vi "Requests.vi"(8 "error in (no error)":errorcluster, 9 "write enable":bool=TRUE, 10 "msg":refnum<queue>, 11 "SP in":refnum<class "Save messages PGserver.lvclass">) -> (0 "error out":errorcluster, 1 "queue deleted":bool, 3 "SP out":refnum<class "Save messages PGserver.lvclass">)   [LabVIEW 2019, in "Save messages PGserver.lvclass"]
uses:
  Save messages PGserver.lvclass
  Save messages PGserver.lvclass/Save messages PGserver.ctl
  PostgreSQL2LabVIEW/libpqlv/src/PQresultErrorMessage.vi
  PostgreSQL2LabVIEW/libpqUtility/src/PQclear.vi
  PostgreSQL2LabVIEW/libpqlv/src/PQsendQuery.vi
  PostgreSQL2LabVIEW/libpqlv/src/PQgetResult.vi
  PostgreSQL2LabVIEW/libpqlv/src/PQresultStatus.vi
  PostgreSQL2LabVIEW/libpqlv/src/PQclear.vi
  PostgreSQL2LabVIEW/libpqUtility/libpqutility.lvlib
  PostgreSQL2LabVIEW/libpqUtility64/libpqutility64.lvlib
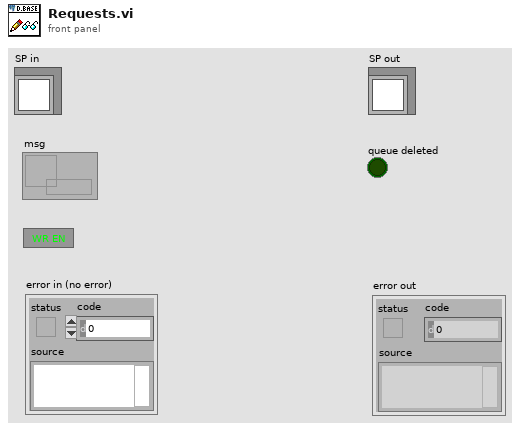
[diagram p1: front panel]
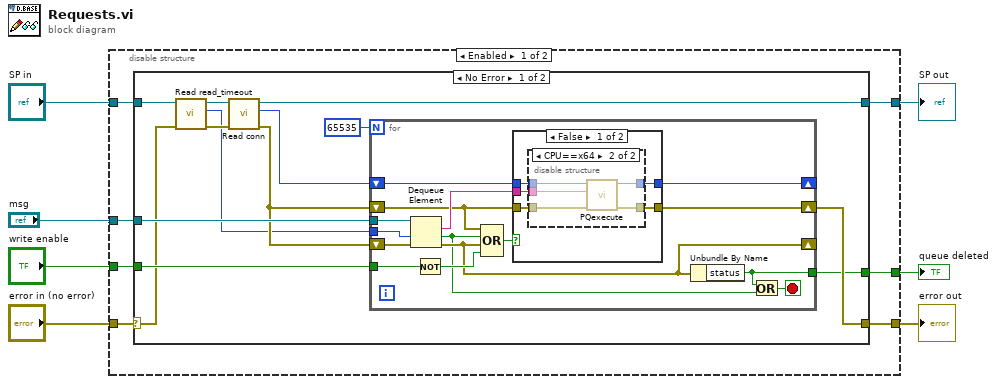
[diagram p0: block diagram]
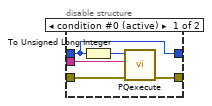
[diagram p2: hidden frame]
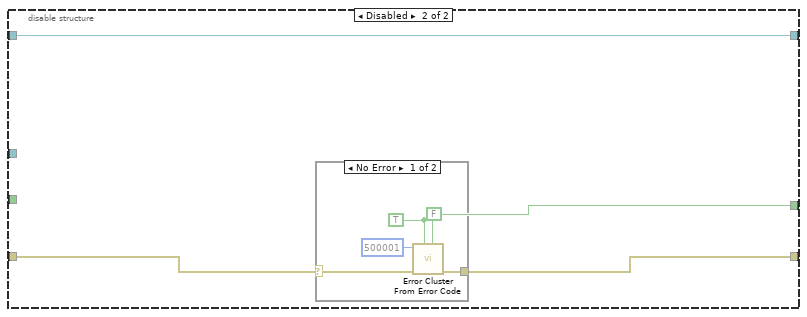
[diagram p5: hidden frame]
diagram:
  n1 = disable-structure shown="Enabled" {
    disable-tunnel: "error in (no error)" -> [w14 w63]
    disable-tunnel: [w13 w64] -> w6
    disable-tunnel: "SP in" -> [w12 w65]
    disable-tunnel: [w11 w65] -> w4
    disable-tunnel: "write enable" -> [w10 _]
    disable-tunnel: "msg" -> [w9 _]
    disable-tunnel: [w8 FALSE ("status")] -> w1
    frame Enabled {
      n2 = case shown="No Error" w14 {
        selector: w14 -> [w16 w61]
        tunnel: [w27 w61] -> w13
        tunnel: [w24 w60] -> w11
        tunnel: w12 -> [w17 w60]
        tunnel: w10 -> [w26 _]
        tunnel: w9 -> [w23 _]
        tunnel: [w21 _] -> w8
        frame No Error {
          n3 = call "Read read_timeout.vi"("error in (no error)"=w16, "SP in"=w17) -> ("error out"=w19:errorcluster, "read_timeout"=w15:i32, "SP out"=w18:refnum<class "Save messages PGserver.lvclass">)  [unwired: 7 in]
          n4 = call "Read conn.vi"("error in (no error)"=w19, "SP in"=w18) -> ("error out"=w20:errorcluster, "conn"=w25:u64, "SP out"=w24:refnum<class "Save messages PGserver.lvclass">)  [unwired: 7 in]
          n5 = for {
            N: 65535 -> [_]
            tunnel: w23 -> [w40]
            tunnel: w15 -> [w34]
            shift-right: [w39] -> _
            shift-left: w25 -> [w41]
            tunnel: w26 -> [w38]
            shift-right: [w42] -> w27
            shift-left: w20 -> [w32]
            tunnel: [w29] -> w21
            shift-right: [w30] -> _
            shift-left: w20 -> [w33]
            stop <- w31 stop-if-true
            n6 = Dequeue Element(queue=w40, timeout in ms (-1)=w34, error in (no error)=w33) -> (element=w35:string, timed out?=w28:bool, error out=w30:errorcluster)  [unwired: 1 out]
            n7 = Not(x=w38) -> (.not. x?=w36:bool)
            n8 = Compound Arithmetic op=OR(w32, w28, w30, w36) -> (w37:bool)
            n9 = case shown="False" w37 {
              tunnel: w32 -> [w47 w59]
              tunnel: w41 -> [w46 w58]
              tunnel: [w44 w59] -> w42
              tunnel: w35 -> [w43 _]
              tunnel: [w45 w58] -> w39
              frame False {
                n10 = disable-structure shown="CPU==x64" {
                  disable-tunnel: w47 -> [w52 w57]
                  disable-tunnel: w46 -> [w48 w56]
                  disable-tunnel: [w48 w55] -> w45
                  disable-tunnel: [w51 w54] -> w44
                  disable-tunnel: w43 -> [w50 w53]
                  frame condition #0 (active) {
                    n11 = To Unsigned Long Integer(number=w48) -> (unsigned 32bit integer=w49:u32)
                    n12 = call "PQexecute.vi"("error in"=w52, "SQL querry"=w50, "conn"=w49) -> ("error out"=w51:errorcluster)  [unwired: 7 in, 1 out]
                  }
                  frame condition #1 {
                    n13 = call "PQexecute.vi"("error in"=w57, "SQL querry"=w53, "conn"=w56) -> ("error out"=w54:errorcluster, "conn_out"=w55:u64)  [unwired: 7 in]
                  }
                }
              }
              frame True {
              }
            }
            n14 = Unbundle By Name(w30) -> ("status"=w29:bool)
            n15 = Or(x=w29, y=w28) -> (x .or. y?=w31:bool)
          }
        }
        frame Error {
        }
      }
    }
    frame Disabled {
      n16 = case shown="No Error" w63 {
        selector: w63 -> [w66 w70]
        tunnel: [w67 w70] -> w64
        frame No Error {
          w68 = TRUE ("show call chain? (False)")
          n17 = call <vilib>:"Error Cluster From Error Code.vi"("is warning? (False)"=w68, "show call chain? (False)"=w68, "error in (no error)"=w66, "error code (0)"=500001) -> ("error out"=w67:errorcluster)  [unwired: 5 in]
        }
        frame Error {
        }
      }
    }
  }
  "error out" <- w6
  "SP out" <- w4
  "queue deleted" <- w1
